vi "DAQ6363_PulseGenAcq.vi"(6 "HaltRef":refnum<vi>, 7 "CntTaskIn":refnum<k21>, 8 "error in (no error)":errorcluster caption="entrée d'erreur (pas d'erreur)", 9 "MWTaskIn":refnum<k21>, 10 "APDTaskIn":refnum<k21>, 11 "LaserTaskIn":refnum<k21>) -> (0 "error out":errorcluster caption="sortie d'erreur", 1 "MWTaskOut":refnum<k21>, 2 "APDTaskOut":refnum<k21>, 3 "LaserTaskOut":refnum<k21>, 4 "Counts Out":u32 caption="CountsOut", 5 "CntTaskOut":refnum<k21>)   [LabVIEW 2019]
uses:
  <vilib>/DAQmx/read.llb/DAQmx Read (Counter U32 1Chan 1Samp).vi
  <userlib>/GenProg/ReadValByRefBool.vi
  <vilib>/DAQmx/miscellaneous.llb/DAQmx Fill In Error Info.vi
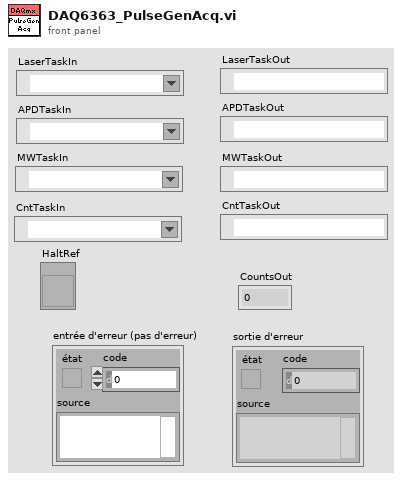
[diagram p1: front panel]
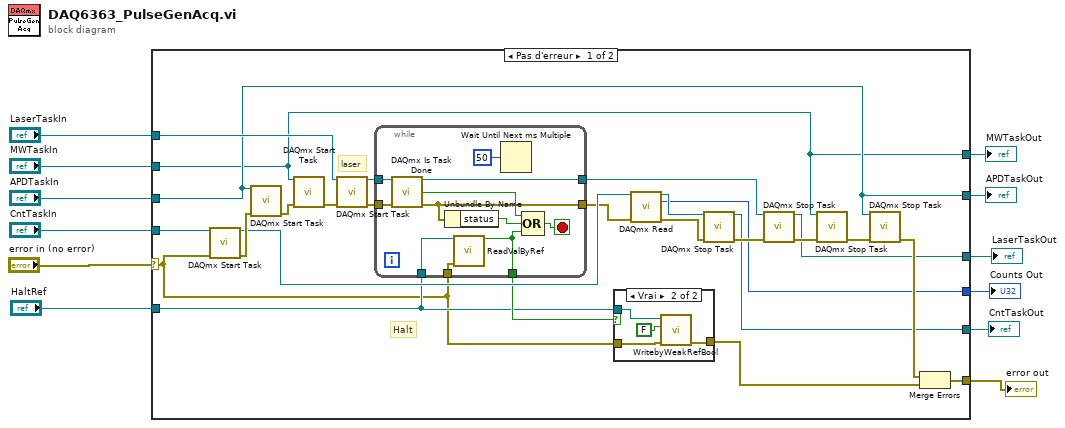
[diagram p0: block diagram]
diagram:
  n1 = case shown="Pas d'erreur" "error in (no error)" {
    selector: "error in (no error)" -> [w21 w55]
    tunnel: [w20 w55] -> w10
    tunnel: "LaserTaskIn" -> [w23 w59]
    tunnel: "CntTaskIn" -> [w24 w56]
    tunnel: "HaltRef" -> [w22 _]
    tunnel: "MWTaskIn" -> [w13 w57]
    tunnel: "APDTaskIn" -> [w14 w58]
    tunnel: [w17 _] -> w5
    tunnel: [w16 w59] -> w4
    tunnel: [w15 w56] -> w3
    tunnel: [w14 w58] -> w2
    tunnel: [w13 w57] -> w1
    frame No Error {
      # "laser"
      # "Halt"
      n2 = call <vilib>:"DAQmx Start Task.vi"("task/channels in"=w24, "error in"=w21) -> ("task out"=w33:refnum<k21>, "error out"=w35:errorcluster)  [unwired: 12 in]
      n3 = call <vilib>:"DAQmx Start Task.vi"("task/channels in"=w14, "error in"=w35) -> ("error out"=w36:errorcluster)  [unwired: 12 in, 1 out]
      n4 = call <vilib>:"DAQmx Start Task.vi"("task/channels in"=w13, "error in"=w36) -> ("error out"=w37:errorcluster)  [unwired: 12 in, 1 out]
      n5 = call <vilib>:"DAQmx Start Task.vi"("task/channels in"=w23, "error in"=w37) -> ("task out"=w38:refnum<k21>, "error out"=w34:errorcluster)  [unwired: 12 in]
      n6 = while {
        tunnel: w38 -> [w54]
        tunnel: w34 -> [w53]
        tunnel: [w50] -> w32
        tunnel: [w51] -> w29
        tunnel: w22 -> [w46]
        tunnel: w21 -> [w45]
        tunnel: [w44] -> w25
        stop <- w52 stop-if-true
        n7 = call <vilib>:"DAQmx Is Task Done.vi"("task/channels in"=w54, "error in"=w53) -> ("task out"=w51:refnum<k21>, "task done?"=w47:bool, "error out"=w50:errorcluster)  [unwired: 11 in]
        n8 = Unbundle By Name(w50) -> ("status"=w49:bool)
        n9 = call-poly <userlib>:"ReadValByRef.vi"("Control Ref"=w46, "error in"=w45) -> ("Valeur"=w44:bool)  [unwired: 12 in, 1 out]
        n10 = Wait Until Next ms Multiple(millisecond multiple=u32 50 ("n millisecondes")) -> ()  [unwired: 1 out]
        n11 = Compound Arithmetic op=OR(w47, w49, w44) -> (w52:bool)
      }
      n12 = case shown="Vrai" w25 {
        tunnel: w22 -> [_ w43]
        tunnel: [w39 w41] -> w18
        tunnel: w21 -> [w39 w40]
        frame False {
        }
        frame True {
          n13 = call <userlib>:"WritebyWeakRefBool.vi"("error in"=w40, "Valeur"=FALSE, "Control Ref"=w43) -> ("error out"=w41:errorcluster)  [unwired: 8 in]
        }
      }
      n14 = call-poly <vilib>:"DAQmx Read.vi"("task/channels in"=w33, "error in"=w32) -> ("task out"=w30:refnum<k21>, "data"=w17:u32, "error out"=w31:errorcluster)  [unwired: 11 in]
      n15 = call <vilib>:"DAQmx Stop Task.vi"("task/channels in"=w30, "error in"=w31) -> ("task out"=w15:refnum<k21>, "error out"=w28:errorcluster)  [unwired: 12 in]
      n16 = call <vilib>:"DAQmx Stop Task.vi"("task/channels in"=w29, "error in"=w28) -> ("task out"=w16:refnum<k21>, "error out"=w27:errorcluster)  [unwired: 12 in]
      n17 = call <vilib>:"DAQmx Stop Task.vi"("task/channels in"=w13, "error in"=w27) -> ("error out"=w26:errorcluster)  [unwired: 12 in, 1 out]
      n18 = call <vilib>:"DAQmx Stop Task.vi"("task/channels in"=w14, "error in"=w26) -> ("error out"=w19:errorcluster)  [unwired: 12 in, 1 out]
      n19 = Merge Errors(w19, w18) -> (w20:errorcluster)
    }
    frame Error {
    }
  }
  "error out" <- w10
  "LaserTaskOut" <- w4
  "Counts Out" <- w5
  "MWTaskOut" <- w1
  "CntTaskOut" <- w3
  "APDTaskOut" <- w2
